vi "Return First Values.vi"(1 "Reset":bool, 2 "Values":dbl) -> (0 "First Value":dbl)   [LabVIEW 2018]
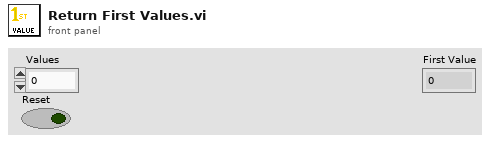
[diagram p1: front panel]
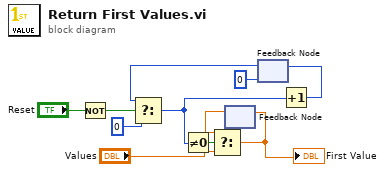
[diagram p0: block diagram]
diagram:
  n1 = Not(x="Reset") -> (.not. x?=w7:bool)
  n2 = feedback #1() -> (w6:dbl)  [unwired: 1 in]
  n3 = feedback #2(0) -> (w2:i32)
  n4 = Select(t=w2, s=w7, f=0) -> (s? t:f=w1:i32)
  n5 = Not Equal To 0?(x=w1) -> (x != 0?=w5:bool)
  n6 = Select(t=w6, s=w5, f="Values") -> (s? t:f=w4:dbl)
  "First Value" <- w4
  n7 = feedback-in #1(w4) -> ()
  n8 = Increment(x=w1) -> (x+1=w10:i32)
  n9 = feedback-in #2(w10) -> ()
